vi "Ping - .NET.vi"(8 "error in (no error)":errorcluster, 9 "timeout":i32=100, 10 "SetSize":i32=32, 11 "IP/Address":string="127.0.0.1") -> (0 "error out":errorcluster, 2 "RoundtripTime":i64, 3 "Status":i32(ring) items=["Success"=0, "DestinationNetworkUnreachable"=11002, "DestinationHostUnreachable"=11003, "DestinationProhibited, DestinationProtocolUnreachable"=11004, "DestinationPortUnreachable"=11005, "NoResources"=11006, "BadOption"=11007, "HardwareError"=11008, "PacketTooBig"=11009, "TimedOut"=11010, "BadRoute"=11012, "TtlExpired"=11013, "TtlReassemblyTimeExceeded"=11014, "ParameterProblem"=11015, "SourceQuench"=11016, "BadDestination"=11018, "DestinationUnreachable"=11040, "TimeExceeded"=11041, "BadHeader"=11042, "UnrecognizedNextHeader"=11043, "IcmpError"=11044, "DestinationScopeMismatch"=11045, "Unknown"=-1])   [LabVIEW 2020]
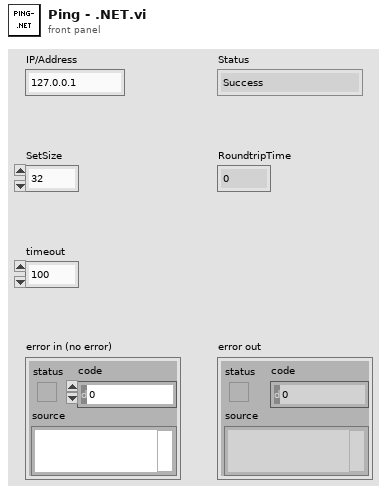
[diagram p1: front panel]
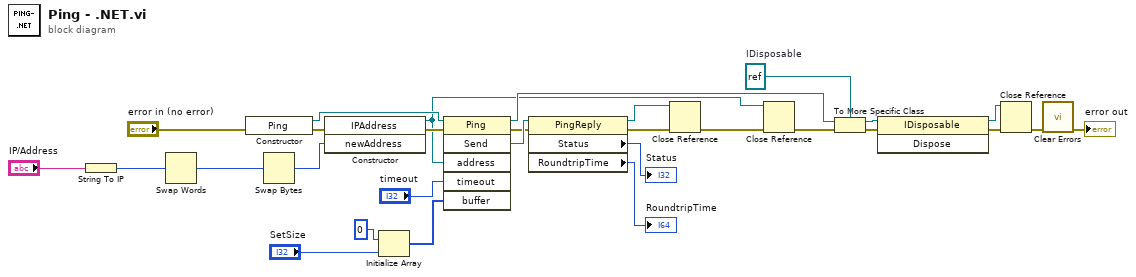
[diagram p0: block diagram]
diagram:
  w11 = refnum<k24> refnum  # IDisposable
  n1 = String To IP(1:"IP/Address") -> (0:w15:u32)
  n2 = Swap Words(1:w15) -> (0:w13:u32)
  n3 = constructor class="Ping"(error in="error in (no error)") -> (reference out=w20:refnum<k24>, error out=w17:errorcluster)  [unwired: 2 in, 1 out]
  n4 = Swap Bytes(anything=w13) -> (byte swapped=w14:u32)
  n5 = constructor class="IPAddress"(error in=w17, "newAddress"=w14) -> (reference out=w7:refnum<k24>, error out=w16:errorcluster)  [unwired: 2 in, 2 out]
  n6 = Initialize Array(u8 0, "SetSize") -> (w19:u8[])
  n7 = invoke class="Ping" method="Send"(reference=w20, error in=w16, "address"=w7, "timeout"="timeout", "buffer"=w19) -> (reference out=w12:refnum<k24>, error out=w21:errorcluster, "Send"=w22:refnum<k24>)  [unwired: 1 in, 3 out]
  n8 = property class="PingReply"(reference=w22, error in=w21) -> (reference out=w10:refnum<k24>, error out=w9:errorcluster, "Status"=→"Status":i32, "RoundtripTime"=→"RoundtripTime":i64)
  n9 = Close Reference(reference=w10, error in (no error)=w9) -> (error out=w8:errorcluster)
  n10 = Close Reference(reference=w7, error in (no error)=w8) -> (error out=w6:errorcluster)
  n11 = To More Specific Class(target class=w11, reference=w12, error in=w6) -> (specific class reference=w5:refnum<k24>, error out=w4:errorcluster)
  n12 = invoke class="IDisposable" method="Dispose"(reference=w5, error in=w4) -> (reference out=w2:refnum<k24>, error out=w3:errorcluster)  [unwired: 1 in, 1 out]
  n13 = Close Reference(reference=w2, error in (no error)=w3) -> (error out=w1:errorcluster)
  n14 = call <vilib>:"Clear Errors.vi"("error in (no error)"=w1) -> ("error out"=→"error out":errorcluster)  [unwired: 5 in, 1 out]
